vi "Array.Search for Item Based on Pattern.vi"(7 "Patterns":string[](array[string]), 10 "Pattern":string, 11 "List":string[](array[string])) -> (2 "Index":i32, 3 "Found Item":string, 5 "Found":bool)   [LabVIEW 2018]
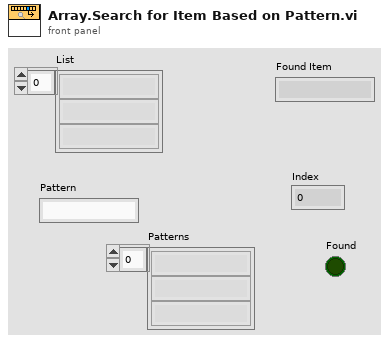
[diagram p1: front panel]
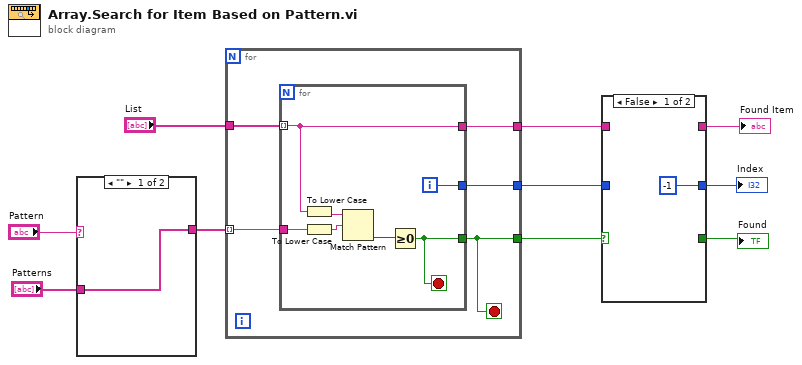
[diagram p0: block diagram]
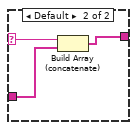
[diagram p2: hidden frame]
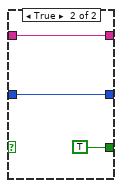
[diagram p3: hidden frame]
diagram:
  n1 = case shown="\"\"" "Pattern" {
    selector: "Pattern" -> [_ w12]
    tunnel: "Patterns" -> [w11 w14]
    tunnel: [w11 w13] -> w3
    frame "" {
    }
    frame Default {
      n2 = Build Array (concatenate)(w12, w14) -> (w13:string[])
    }
  }
  n3 = for {
    tunnel: [w15] -> w10
    tunnel: [w19] -> w9
    tunnel: [w18] -> w8
    tunnel: "List" -> [w17]
    tunnel: w3 -> [w16] mode=indexing
    stop <- w15 stop-if-true
    n4 = for {
      tunnel: w17 -> [w22] mode=indexing
      tunnel: w16 -> [w24]
      tunnel: [w22] -> w18
      tunnel: [w21] -> w15
      tunnel: [w20] -> w19
      i -> [w20]
      stop <- w21 stop-if-true
      n5 = To Lower Case(string=w22) -> (all lower case string=w26:string)
      n6 = To Lower Case(string=w24) -> (all lower case string=w25:string)
      n7 = Match Pattern(string=w26, regular expression=w25) -> (offset past match=w23:i32)  [unwired: 1 in, 3 out]
      n8 = Greater Or Equal To 0?(x=w23) -> (x >= 0?=w21:bool)
    }
  }
  n9 = case shown="False" w10 {
    tunnel: w9 -> [_ w29]
    tunnel: w8 -> [_ w30]
    tunnel: [_ w30] -> w7
    tunnel: [-1 w29] -> w6
    tunnel: [_ TRUE] -> w1
    frame False {
    }
    frame True {
    }
  }
  "Index" <- w6
  "Found Item" <- w7
  "Found" <- w1
